vi "test_GetItemInfosFromProjectFile_HierarchyExampleProject.vi"() -> (3 "Pass?":bool)   [LabVIEW 2019, in "Tests.SolutionBuilder.lvlib"]
uses:
  Tests.SolutionBuilder.lvlib
  SolutionBuilder/SolutionBuilder.lvclass
  SolutionBuilder/ProjectItem/ProjectItem.lvclass
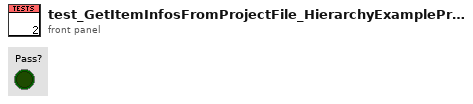
[diagram p1: front panel]
types:
  T1 = typedef "SolutionBuilder.lvlib/SolutionBuilder.lvclass/ProjectItemMap.ctl" = map{path, refnum<class "ProjectItem.lvclass">[]}
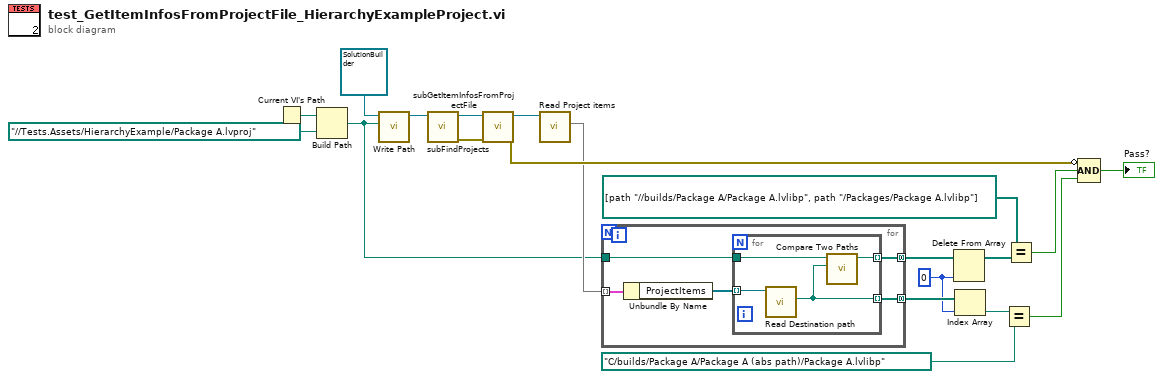
[diagram p0: block diagram]
diagram:
  w4 = 0 ("index")
  n1 = Current VI's Path() -> (path=w17:path)
  n2 = Build Path(base path=w17, name or relative path=path "../../Tests.Assets/HierarchyExample/Package A.lvproj" ("Path")) -> (appended path=w10:path)
  n3 = call "Write Path.vi"("Path"=w10, "SolutionBuilder in"=refnum<class "SolutionBuilder.lvclass"> refnum) -> ("SolutionBuilder out"=w19:refnum<class "SolutionBuilder.lvclass">)  [unwired: 9 in]
  n4 = call "subFindProjects.vi"("SolutionBuilder in"=w19) -> ("error out"=w15:errorcluster, "SolutionBuilder out"=w18:refnum<class "SolutionBuilder.lvclass">)  [unwired: 9 in]
  n5 = call "subGetItemInfosFromProjectFile.vi"("error in (no error)"=w15, "SolutionBuilder in"=w18) -> ("error out"=w14:errorcluster, "SolutionBuilder out"=w12:refnum<class "SolutionBuilder.lvclass">)  [unwired: 8 in]
  n6 = call "Read Project items.vi"("SolutionBuilder in"=w12) -> ("Project items"=w11:T1)  [unwired: 9 in, 1 out]
  n7 = for {
    tunnel: w11 -> [w25] mode=indexing
    tunnel: [w23] -> w7 mode=concatenating
    tunnel: w10 -> [w22]
    tunnel: [w21] -> w5 mode=concatenating
    n8 = Unbundle By Name(w25) -> ("ProjectItems"=w24:refnum<class "ProjectItem.lvclass">[])
    n9 = for {
      tunnel: w24 -> [w29] mode=indexing
      tunnel: [w27] -> w23 mode=indexing
      tunnel: w22 -> [w28]
      tunnel: [w26] -> w21 mode=indexing
      n10 = call "Read Destination path.vi"("ProjectItem in"=w29) -> ("Destination path"=w26:path)  [unwired: 9 in, 1 out]
      n11 = call <vilib>:"Compare Two Paths.vi"("Path 2"=w26, "Path 1"=w28) -> ("Relative Path from 1 to 2"=w27:path)  [unwired: 6 in, 3 out]
    }
  }
  n12 = Delete From Array(array=w7, index=w4) -> (array with subset deleted=w6:path[])  [unwired: 1 in, 1 out]
  n13 = Index Array(array=w5, index=w4) -> (element=w3:path)
  n14 = Equal?(x=w3, y=path "C:/builds/Package A/Package A (abs path)/Package A.lvlibp" ("Relative Path from 1 to 2")) -> (x = y?=w1:bool)
  n15 = Equal?(x=path[] [path "../../builds/Package A/Package A.lvlibp", path "../Packages/Package A.lvlibp"] ("y"), y=w6) -> (x = y?=w8:bool)
  n16 = Compound Arithmetic op=AND(invert w14, w8, w1) -> (→"Pass?":bool)
